vi "RN_Motor_Grad_Drehen_NEMA17.vi"(6 "error in":errorcluster, 7 "Drehwinkel (°)":dbl=90.0 min=0.0 max=58982.4 step=0.9 format="%#.1f", 8 "Motorwahl":string(combo)="#rmd\u0000\u0000", 9 "VISA resource name in":refnum<visa-resource-name>="COM5") -> (0 "error out":errorcluster, 2 "Gesendeter Code":string, 3 "VISA resource name out":refnum<visa-resource-name>="COM5")   [LabVIEW 2014]
doc: "VI zum Drehen der Motoren der RN-Motorsteuerung um eine selbstdefinierte Anzahl von Schritten;\n\nDie Eingabe erfolgt in Grad ()\n\nStandardwert: 360 = 400 Schritte\n\nmögliche Werte: 0,9 - 58982,4"
panel:
  out "x*y":dbl=1361.9834710743803
  in  "Steuercode":string="z"
  in  "Kennung - RN-Motorsteuerung":string="#rm"
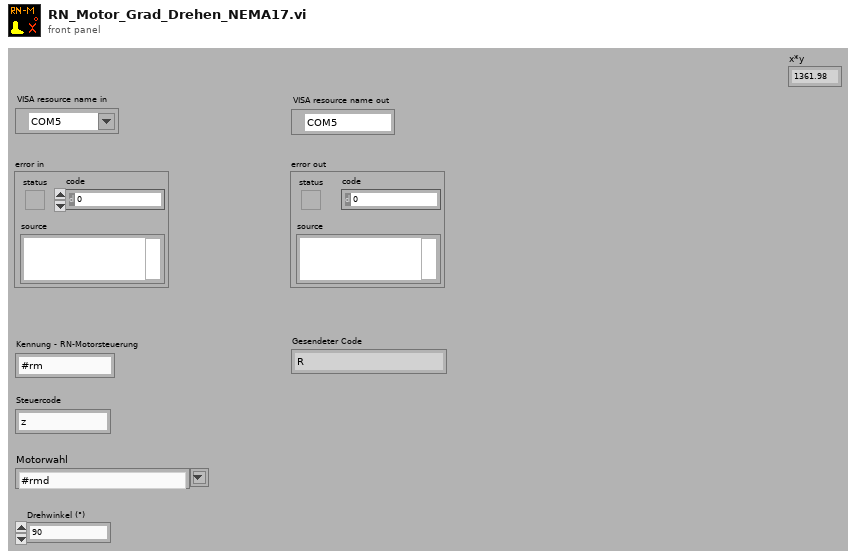
[diagram p1: front panel]
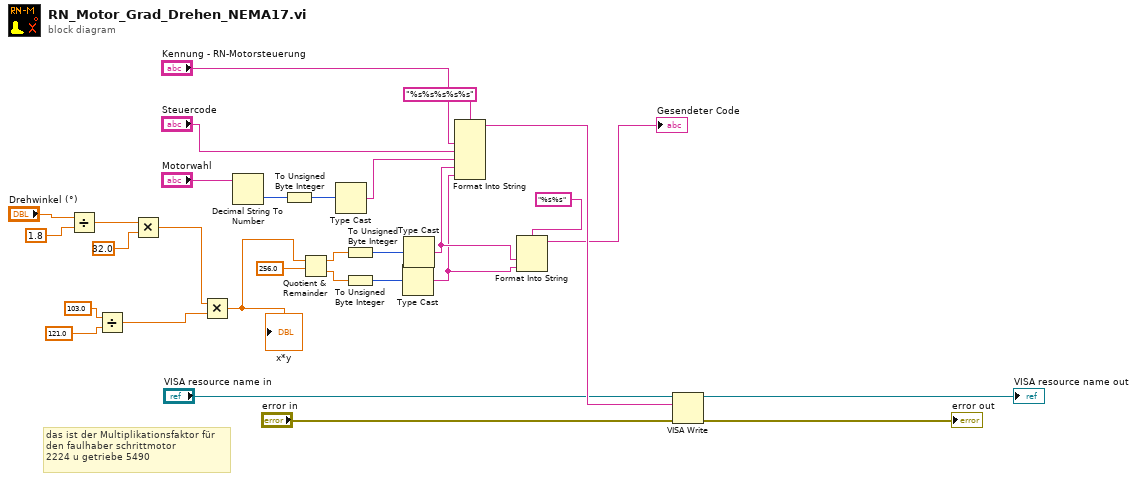
[diagram p0: block diagram]
diagram:
  # "das ist der Multiplikationsfaktor für \nden faulhaber schrittmotor \n2224 u getriebe 5490"
  n1 = Divide(x="Drehwinkel (°)", y=1.8) -> (x/y=w11:dbl)
  n2 = Divide(x=103.0 ("y"), y=121.0) -> (x/y=w3:dbl)
  n3 = Multiply(x=w11, y=32.0) -> (x*y=w2:dbl)
  n4 = Multiply(x=w2, y=w3) -> (x*y=w1:dbl)
  "x*y" <- w1
  n5 = Decimal String To Number(string="Motorwahl") -> (number=w29:i32)  [unwired: 2 in, 1 out]
  n6 = To Unsigned Byte Integer(number=w29) -> (unsigned 8bit integer=w28:u8)
  n7 = Quotient & Remainder(x=w1, y=256.0) -> (x-y*floor(x/y)=w14:dbl, floor(x/y)=w16:dbl)
  n8 = Type Cast(x=w28) -> (*(type *) &x=w25:string)  [unwired: 1 in]
  n9 = To Unsigned Byte Integer(number=w14) -> (unsigned 8bit integer=w17:u8)
  n10 = To Unsigned Byte Integer(number=w16) -> (unsigned 8bit integer=w15:u8)
  n11 = Type Cast(x=w15) -> (*(type *) &x=w8:string)  [unwired: 1 in]
  n12 = Type Cast(x=w17) -> (*(type *) &x=w9:string)  [unwired: 1 in]
  n13 = Format Into String(format string="%s%s%s%s%s", "Kennung - RN-Motorsteuerung", "Steuercode", w25, w9, w8) -> (resulting string=w24:string)  [unwired: 2 in, 1 out]
  n14 = Format Into String(format string="%s%s", w9, w8) -> (resulting string=→"Gesendeter Code":string)  [unwired: 2 in, 1 out]
  n15 = VISA Write(VISA resource name="VISA resource name in", write buffer=w24, error in (no error)="error in") -> (VISA resource name out=→"VISA resource name out":refnum<visa-resource-name>, error out=→"error out":errorcluster)  [unwired: 1 out]
